vi "Measurement Core.vi"(8 "error in (no error)":errorcluster, 11 "ModSweep in":refnum<class "ModSweep.lvclass">) -> (0 "error out":errorcluster, 3 "ModSweep out":refnum<class "ModSweep.lvclass">)   [LabVIEW 2018]
uses:
  ModSweep.lvclass
  Plugins/TestStand API Tools (TSAT).lvlibp/Step Actions/TSAT Step Actions.lvlib
  Plugins/Measurement Interface.lvlibp/Measurement Interface.lvclass
  C:/Sequence Automation/Plugins/Measurements/Servo MSMT.lvlibp/Servo MSMT.lvclass
  C:/Sequence Automation/Plugins/Measurement Interface.lvlibp/Measurement Interface.lvclass
  C:/Sequence Automation/Plugins/FPF.lvlibp/Factory Plugin Framework.lvclass
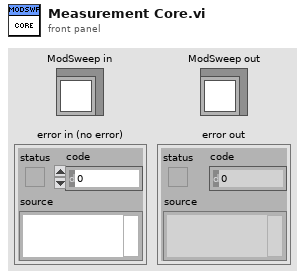
[diagram p1: front panel]
types:
  T1 = typedef "TestStand API Tools (TSAT).lvlibp/TSAT Evaluation Actions.lvlib/TSAT Evaluation.ctl" = cluster{"Test Name":string, "Pin":string, "Units":string, "SI Scaling":T2, "Test Number":i32, "Published Data Id":string, "Low Limit":dbl, "High Limit":dbl, "Export Data Location":string, "Software Bin":i64, "Evaluation Type":T3, "Test Data Source":string}
  T2 = typedef "TestStand API Tools (TSAT).lvlibp/TSAT Evaluation Actions.lvlib/TSAT Eval SI Unit Scaling.ctl" = i16
  T3 = typedef "TestStand API Tools (TSAT).lvlibp/TSAT Evaluation Actions.lvlib/TSAT Evaluation Type.ctl" = enum16{"Numeric Limit", "Pass/Fail", "None"}
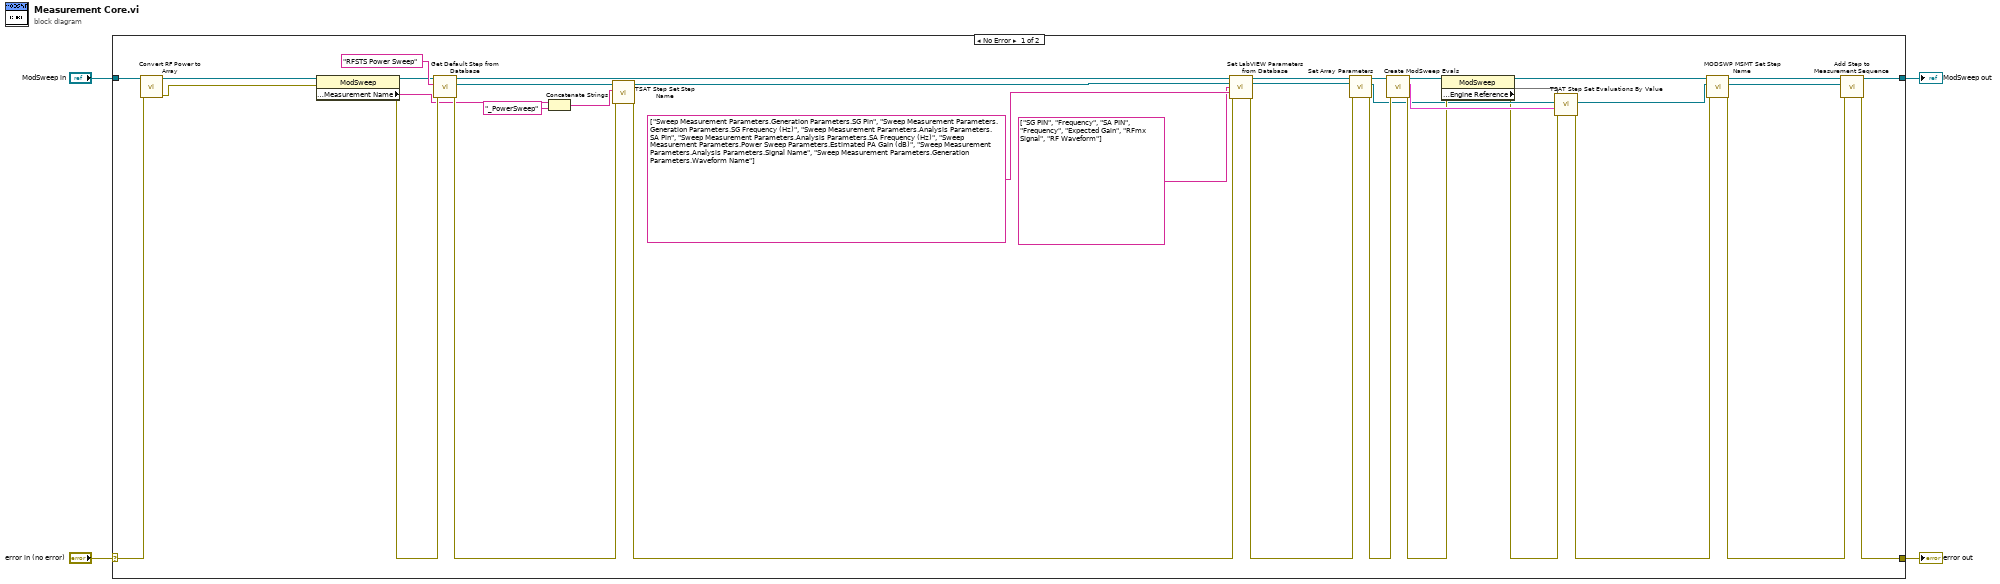
[diagram p0: block diagram]
diagram:
  n1 = case shown="No Error" "error in (no error)" {
    selector: "error in (no error)" -> [w32 w42]
    tunnel: [w20 w42] -> w3
    tunnel: [w19 w41] -> w1
    tunnel: "ModSweep in" -> [w33 w41]
    frame No Error {
      n2 = call "Convert RF Power to Array.vi"("error in (no error)"=w32, "ModSweep in"=w33) -> ("error out"=w31:errorcluster, "ModSweep out"=w5:refnum<class "ModSweep.lvclass">)  [unwired: 8 in]
      n3 = property class="ModSweep"(reference=w5, error in=w31) -> (reference out=w9:refnum<class "ModSweep.lvclass">, error out=w10:errorcluster, "Public Methods:Measurement Name"=w8:string)
      n4 = call "Get Default Step from Database.vi"("error in (no error)"=w10, "Default Step"="RFSTS Power Sweep" ("FileGlobal to Clone"), "Measurement Interface in"=w9) -> ("error out"=w40:errorcluster, "Cloned Step"=w17:refnum<k7>, "Measurement Interface out"=w38:refnum<class "ModSweep.lvclass">)  [unwired: 6 in]
      n5 = Concatenate Strings(w8, "_PowerSweep" ("string")) -> (w7:string)
      n6 = call "TSAT Step Set Step Name.vi"("Error In"=w40, "Name"=w7, "Step In"=w17) -> ("Error Out"=w18:errorcluster, "Step Out"=w16:refnum<k7>)  [unwired: 7 in]
      n7 = call "Set LabVIEW Parameters from Database.vi"("Measurement Interface in"=w38, "Step In"=w16, "Dictionary Keys"=string[] ["SG PIN", "Frequency", "SA PIN", "Frequency", "Expected Gain", "RFmx Signal", "RF Waveform"] ("Local Variable Mapping"), "LabVIEW Parameter Mapping"=string[] ["Sweep Measurement Parameters.Generation Parameters.SG Pin", "Sweep Measurement Parameters.Generation Parameters.SG Frequency (Hz)", "Sweep Measurement Parameters.Analysis Parameters.SA Pin", "Sweep Measurement Parameters.Analysis Parameters.SA Frequency (Hz)", "Sweep Measurement Parameters.Power Sweep Parameters.Estimated PA Gain (dB)", "Sweep Measurement Parameters.Analysis Parameters.Signal Name", "Sweep Measurement Parameters.Generation Parameters.Waveform Name"] ("Local Variable Mapping"), "error in (no error)"=w18) -> ("Measurement Interface out"=w30:refnum<class "ModSweep.lvclass">, "Step Out"=w29:refnum<k7>, "error out"=w35:errorcluster)  [unwired: 8 in]
      n8 = call "Set Array Parameters.vi"("error in (no error)"=w35, "Step In"=w29, "ModSweep in"=w30) -> ("error out"=w34:errorcluster, "Step Out"=w24:refnum<k7>, "ModSweep out"=w28:refnum<class "ModSweep.lvclass">)  [unwired: 6 in]
      n9 = call "Create ModSweep Evals.vi"("error in (no error)"=w34, "ModSweep in"=w28) -> ("error out"=w26:errorcluster, "Array"=w27:T1[], "ModSweep out"=w22:refnum<class "ModSweep.lvclass">)  [unwired: 7 in]
      n10 = property class="ModSweep"(reference=w22, error in=w26) -> (reference out=w14:refnum<class "ModSweep.lvclass">, error out=w23:errorcluster, "Protected Methods:Engine Reference"=w21)
      n11 = call "TSAT Step Set Evaluations By Value.vi"("Error In"=w23, "Evaluation Data"=w27, "Step In"=w24, "Engine In"=w21) -> ("Error Out"=w25:errorcluster, "Step Out"=w12:refnum<k7>)  [unwired: 5 in, 1 out]
      n12 = call "MODSWP MSMT Set Step Name.vi"("error in (no error)"=w25, "Step In"=w12, "ModSweep in"=w14) -> ("error out"=w15:errorcluster, "Step Out"=w11:refnum<k7>, "ModSweep out"=w13:refnum<class "ModSweep.lvclass">)  [unwired: 6 in]
      n13 = call "Add Step to Measurement Sequence.vi"("error in (no error)"=w15, "Step to Add"=w11, "Measurement Interface in"=w13) -> ("error out"=w20:errorcluster, "Measurement Interface out"=w19:refnum<class "ModSweep.lvclass">)  [unwired: 7 in]
    }
    frame Error {
    }
  }
  "error out" <- w3
  "ModSweep out" <- w1
